vi "vision_acquisition_snap(pic).vi"() -> ()   [LabVIEW 2019]
panel:
  in  "click_me_to _stop":bool
  in  "?":bool
  out "image::::":T1(plugin-control)
  # "Click ok button to take a snap"
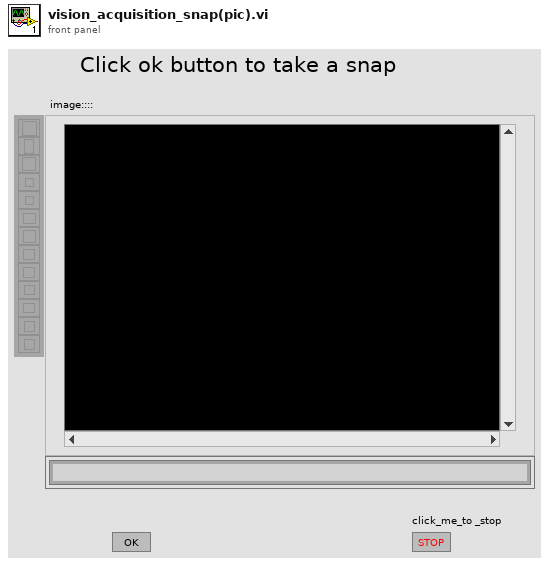
[diagram p1: front panel]
types:
  T1 = typedef "IMAQ Image.ctl" = refnum<image>
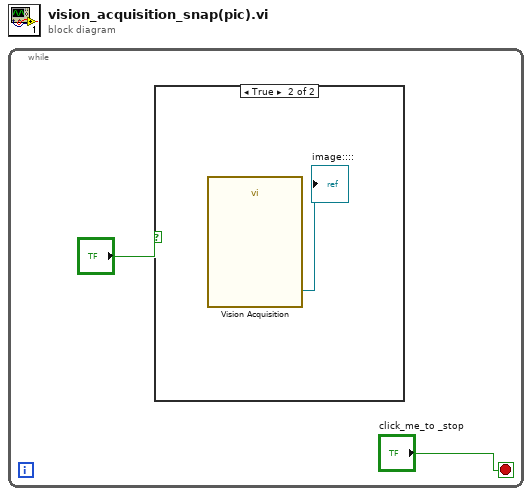
[diagram p0: block diagram]
diagram:
  n1 = while {
    stop <- "click_me_to _stop" stop-if-true
    n2 = case shown="True" "?" {
      frame False {
      }
      frame True {
        n3 = call "Vision Acquisition"() -> ("Image Out"=→"image::::":T1)  [unwired: 26 in, 1 out]
      }
    }
  }
